vi "ADO Command Execute.vi"(8 "error in (no error)":errorcluster, 11 "ADODB._Command In":refnum<k7>) -> (0 "error out":errorcluster, 2 "ADODB._Recordset":refnum<k7>, 3 "ADODB._Command Out":refnum<k7>)   [LabVIEW 2013]
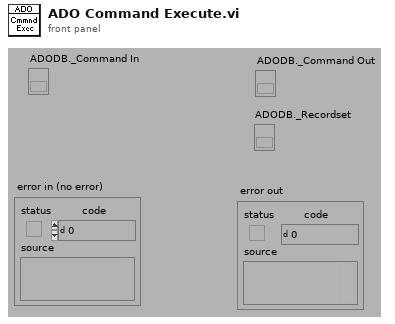
[diagram p1: front panel]
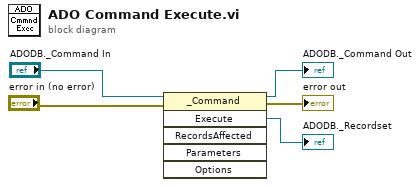
[diagram p0: block diagram]
diagram:
  n1 = invoke class="_Command" method="Execute"(reference="ADODB._Command In", error in="error in (no error)") -> (reference out=→"ADODB._Command Out":refnum<k7>, error out=→"error out":errorcluster, "Execute"=→"ADODB._Recordset":refnum<k7>)  [unwired: 4 in, 3 out]
